vi "Torques_Calc.vi"() -> ()   [LabVIEW 2024]
panel:
  out "Torque 2":dynamicdata(graph) caption="Histogram"
  out "Torque 1":dynamicdata(graph) caption="Histogram"
  out "Torque 2":dbl(graph)
  out "Torque 1":dbl(graph)
  out "Bot Arm":picture
  out "Angle 2":dbl
  out "Angle 1":dbl
  in  "Colors 2":T1={"Base"=16750848, "Link 1"=16764006, "Joint 2"=26316, "Link 2"=6723993, "EOF"=16724787}
  out "GCode Reading":picture
  in  "file (use dialog)":path
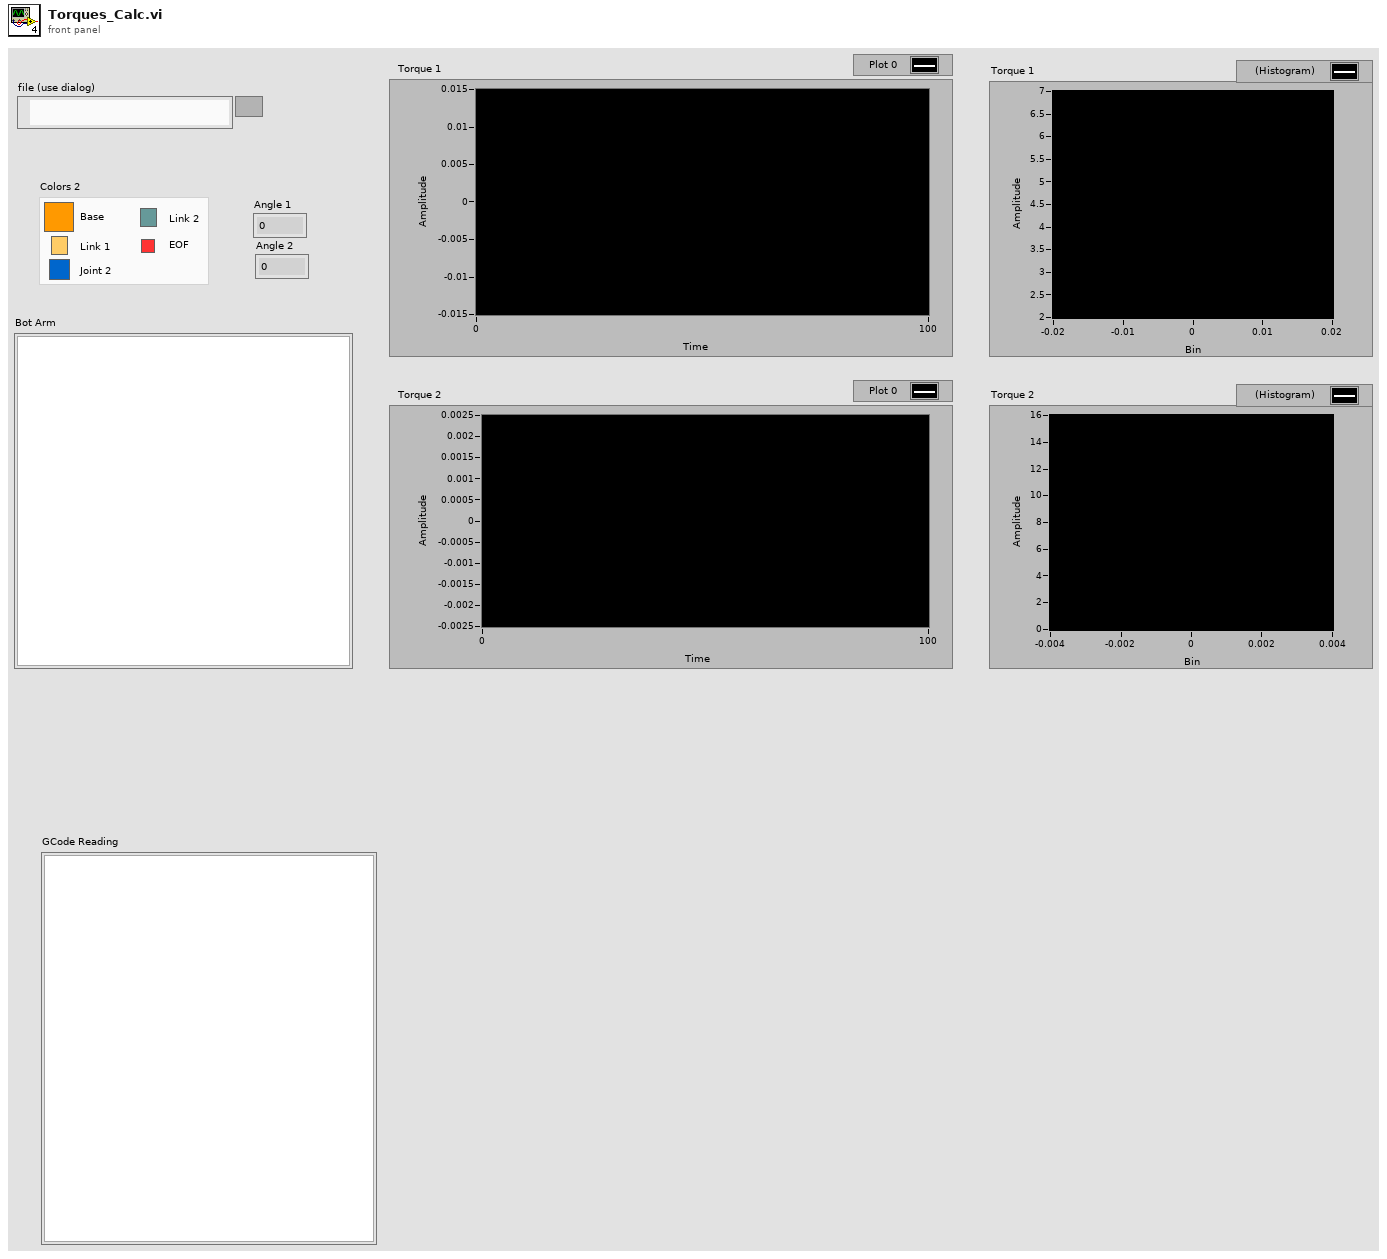
[diagram p1: front panel]
types:
  T1 = cluster{"Base":u32, "Link 1":u32, "Joint 2":u32, "Link 2":u32, "EOF":u32}
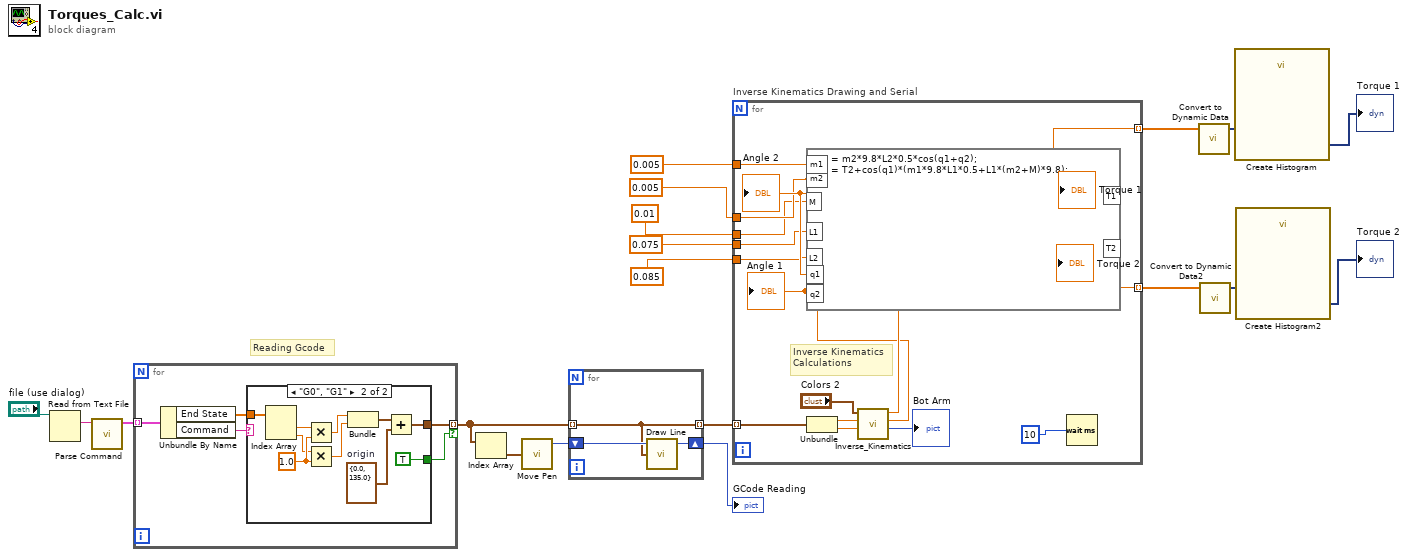
[diagram p0: block diagram]
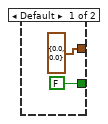
[diagram p2: hidden frame]
diagram:
  # "Reading Gcode"
  n1 = Read from Text File(file (use dialog)="file (use dialog)") -> (text=w18:string)  [unwired: 3 in, 3 out]
  n2 = call "Parse Command.vi"("text"=w18) -> ("cmd amd State"=w17:cluster{"Command":string, "End State":dbl[]}[])  [unwired: 8 in, 2 out]
  n3 = for {
    tunnel: w17 -> [w24] mode=indexing
    tunnel: [w21] -> w13 mode=indexing if=w20
    n4 = Unbundle By Name(w24) -> ("End State"=w22:dbl[], "Command"=w23:string)
    n5 = case shown="\"G0\", \"G1\"" w23 {
      tunnel: w22 -> [_ w36]
      tunnel: [cluster{dbl, dbl} {0.0, 0.0} w33] -> w21
      tunnel: [FALSE TRUE] -> w20
      frame Default {
      }
      frame "G0", "G1" {
        w31 = 1.0 ("y")
        w34 = cluster{dbl, dbl} {0.0, 135.0}  # origin
        n6 = Index Array(array=w36) -> (element #1=w28:dbl, element #2=w27:dbl)  [unwired: 2 in]
        n7 = Multiply(x=w28, y=w31) -> (x*y=w29:dbl)
        n8 = Multiply(x=w27, y=w31) -> (x*y=w30:dbl)
        n9 = Bundle(w29, w30) -> (w35:cluster{dbl, dbl})  [unwired: 1 in]
        n10 = Add(x=w35, y=w34) -> (x+y=w33:cluster{dbl, dbl})
      }
    }
  }
  n11 = Index Array(array=w13) -> (element=w16:cluster{dbl, dbl})  [unwired: 1 in]
  n12 = call <vilib>:"Move Pen.vi"("new position"=w16) -> ("new picture"=w15:picture)  [unwired: 4 in]
  n13 = for {
    shift-right: [w38] -> w14
    shift-left: w15 -> [w39]
    tunnel: w13 -> [w37] mode=indexing
    tunnel: [w37] -> w12 mode=indexing
    n14 = call <vilib>:"Draw Line.vi"("picture"=w39, "end point"=w37) -> ("new picture"=w38:picture)  [unwired: 7 in]
  }
  "GCode Reading" <- w14
  n15 = for "Inverse Kinematics Drawing and Serial" {
    tunnel: w12 -> [w51] mode=indexing
    tunnel: 0.005 -> [w46]
    tunnel: 0.005 -> [w45]
    tunnel: 0.01 -> [w44]
    tunnel: 0.075 -> [w43]
    tunnel: 0.085 -> [w42]
    tunnel: [w41] -> w6 mode=indexing
    tunnel: [w40] -> w3 mode=indexing
    # "Inverse Kinematics\nCalculations"
    n16 = Unbundle(w51) -> (w50:dbl, w49:dbl)
    n17 = call "Inverse_Kinematics.vi"("Numeric in"=w49, "Numeric 3"=w50, "Colors in"="Colors 2") -> ("Picture Out"=→"Bot Arm":picture, "Angle 3"=w47:dbl, "Angle 4"=w48:dbl)  [unwired: 4 in, 2 out]
    "Angle 1" <- w47
    "Angle 2" <- w48
    n18 = formula code="T2 = m2*9.8*L2*0.5*cos(q1+q2);\nT1 = T2+cos(q1)*(m1*9.8*L1*0.5+L1*(m2+M)*9.8);"("m2"=w45, "m1"=w46, "M"=w44, "L1"=w43, "L2"=w42, "q1"=w48, "q2"=w47) -> ("T1"=w41:dbl, "T2"=w40:dbl)
    "Torque 1" <- w41
    "Torque 2" <- w40
    n19 = Wait (ms)(milliseconds to wait=u32 10) -> ()  [unwired: 1 out]
  }
  n20 = call "Convert to Dynamic Data"("Array"=w6) -> ("Dynamic Data Type"=w5:dynamicdata)  [unwired: 3 in]
  n21 = call "Convert to Dynamic Data2"("Array"=w3) -> ("Dynamic Data Type"=w2:dynamicdata)  [unwired: 3 in]
  n22 = call "Create Histogram"("Signal"=w5) -> ("Histogram"=→"Torque 1":dynamicdata)  [unwired: 9 in, 1 out]
  n23 = call "Create Histogram2"("Signal"=w2) -> ("Histogram"=→"Torque 2":dynamicdata)  [unwired: 9 in, 1 out]
